vi "Basic NPL DS Write-Read external.vi"(5 "TimeOut Time (s)":dbl format="%.2f", 6 "error in (no error)":errorcluster, 7 "Server Mode":T2, 8 "Operation Mode":enum16{"Read", "Write", "Write/Read"}(ring), 9 "DataSocketCluster In":T1 {"TimeStamp" format="%.2f"}) -> (0 "error out":errorcluster, 2 "New Data":bool, 3 "DataSocketCluster Out":T1 {"TimeStamp" format="%.2f"})   [LabVIEW 2020]
uses:
  vi Mode external.ctl
  DataSocketCluster external.ctl
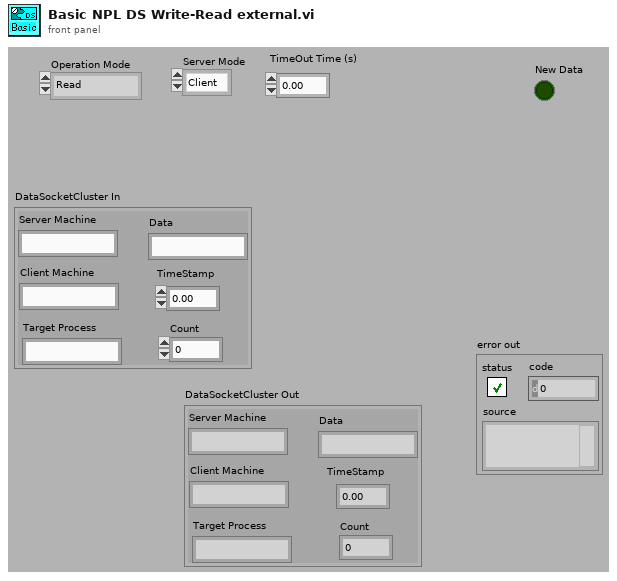
[diagram p1: front panel]
types:
  T1 = typedef "DataSocketCluster external.ctl" = cluster{"Server Machine":string, "Client Machine":string, "Data":string, "TimeStamp":dbl, "Count":i32, "Target Process":string}
  T2 = typedef "vi Mode external.ctl" = enum16{"Client", "Server"}
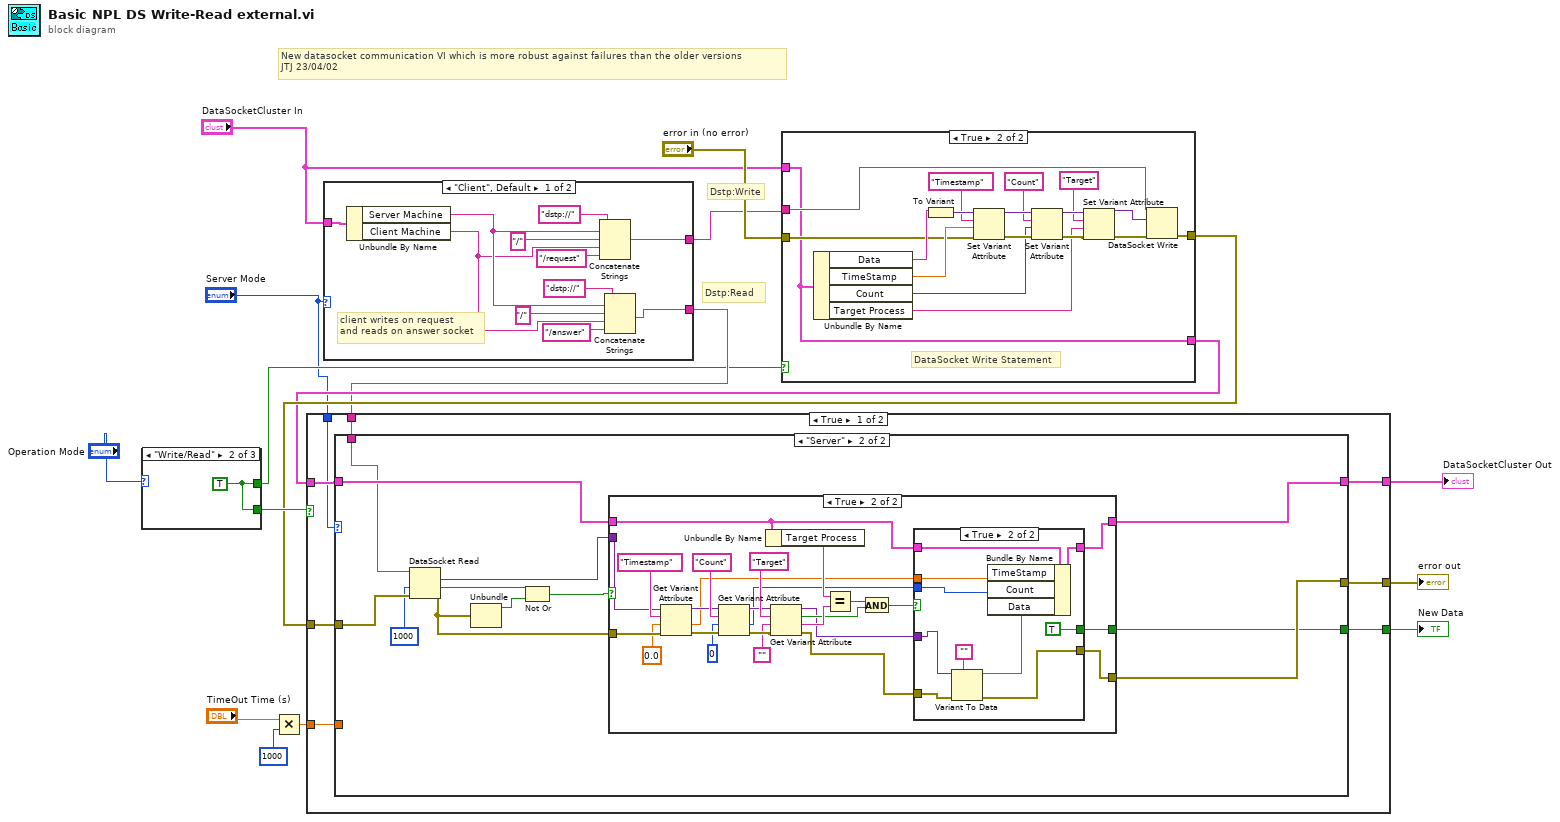
[diagram p0: block diagram]
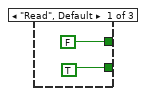
[diagram p2: hidden frame]
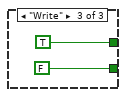
[diagram p3: hidden frame]
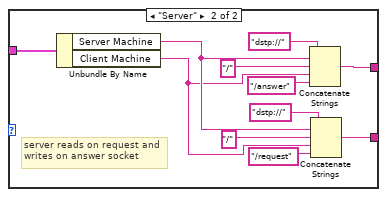
[diagram p5: hidden frame]
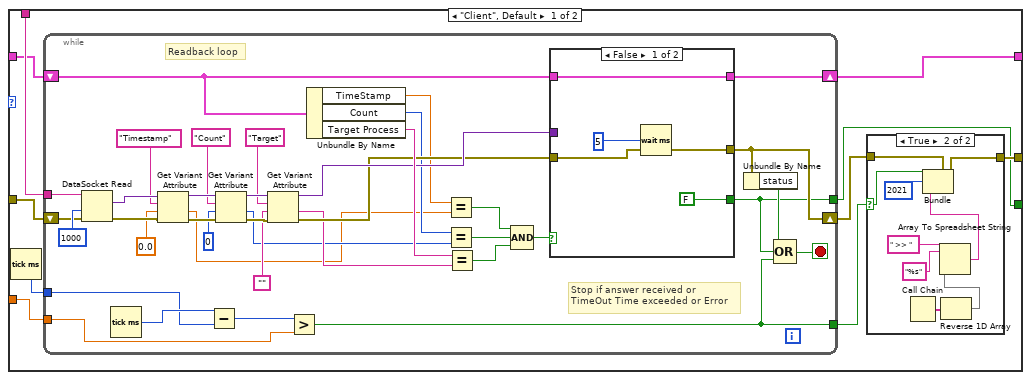
[diagram p6: hidden frame]
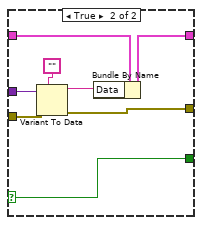
[diagram p7: hidden frame]
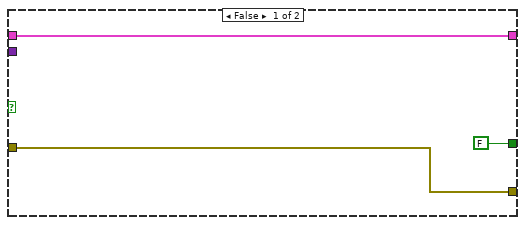
[diagram p9: hidden frame]
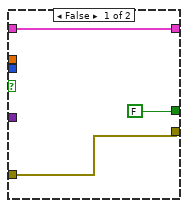
[diagram p10: hidden frame]
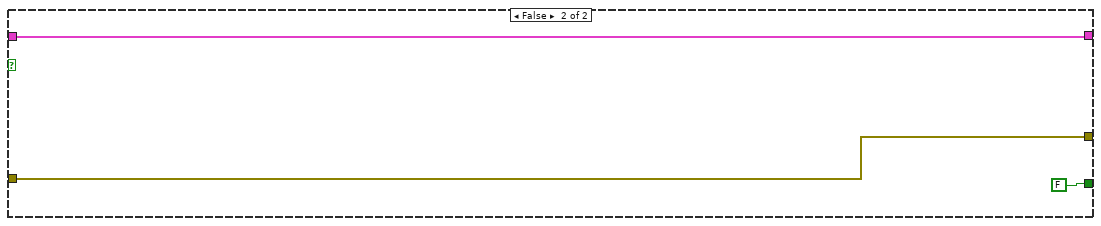
[diagram p11: hidden frame]
diagram:
  # "New datasocket communication VI which is more robust against failures than the older versions\nJTJ 23/04/02"
  # "Dstp:Read"
  # "Dstp:Write"
  n1 = case shown="\"Write/Read\"" "Operation Mode" {
    tunnel: [FALSE w19 TRUE] -> w5
    tunnel: [TRUE w19 FALSE] -> w14
    frame "Read", Default {
    }
    frame "Write/Read" {
      w19 = TRUE
    }
    frame "Write" {
    }
  }
  n2 = Multiply(x="TimeOut Time (s)", y=1000) -> (x*y=w6:dbl)
  n3 = case shown="\"Client\", Default" "Server Mode" {
    tunnel: "DataSocketCluster In" -> [w29 w43]
    tunnel: [w28 w39] -> w10
    tunnel: [w24 w35] -> w11
    frame "Client", Default {
      # "client writes on request\nand reads on answer socket"
      n4 = Unbundle By Name(w29) -> ("Server Machine"=w23:string, "Client Machine"=w22:string)
      n5 = Concatenate Strings("dstp://", w23, "/", w22, "/request") -> (w28:string)
      n6 = Concatenate Strings("dstp://", w23, "/", w22, "/answer") -> (w24:string)
    }
    frame "Server" {
      # "server reads on request and\nwrites on answer socket"
      n7 = Unbundle By Name(w43) -> ("Server Machine"=w34:string, "Client Machine"=w33:string)
      n8 = Concatenate Strings("dstp://", w34, "/", w33, "/answer") -> (w39:string)
      n9 = Concatenate Strings("dstp://", w34, "/", w33, "/request") -> (w35:string)
    }
  }
  n10 = case shown="True" w5 {
    tunnel: "error in (no error)" -> [w45 w49]
    tunnel: [w45 w48] -> w13
    tunnel: [w44 w46] -> w12
    tunnel: "DataSocketCluster In" -> [w44 w46]
    tunnel: w10 -> [_ w47]
    frame False {
    }
    frame True {
      # "DataSocket Write Statement"
      n11 = Unbundle By Name(w46) -> ("Data"=w53:string, "TimeStamp"=w52:dbl, "Count"=w51:i32, "Target Process"=w50:string)
      n12 = To Variant(anything=w53) -> (Variant=w63:variant)
      n13 = Set Variant Attribute(Variant=w63, name="Timestamp", value=w52, error in=w49) -> (Variant out=w62:variant, error out=w56:errorcluster)  [unwired: 1 out]
      n14 = Set Variant Attribute(Variant=w62, name="Count", value=w51, error in=w56) -> (Variant out=w61:variant, error out=w55:errorcluster)  [unwired: 1 out]
      n15 = Set Variant Attribute(Variant=w61, name="Target", value=w50, error in=w55) -> (Variant out=w57:variant, error out=w54:errorcluster)  [unwired: 1 out]
      n16 = DataSocket Write(8:w54, 10:w57, 11:w47) -> (0:w48:errorcluster)  [unwired: 1 in, 2 out]
    }
  }
  n17 = case shown="True" w14 {
    tunnel: w13 -> [w70 w196]
    tunnel: w11 -> [w71 _]
    tunnel: [w68 w197] -> w2
    tunnel: w6 -> [w69 _]
    tunnel: w12 -> [w67 w197]
    tunnel: [w66 w196] -> w9
    tunnel: "Server Mode" -> [w65 _]
    tunnel: [w64 FALSE] -> w4
    frame True {
      n18 = case shown="\"Server\"" w65 {
        tunnel: w71 -> [w81 w146]
        tunnel: w70 -> [w80 w148]
        tunnel: w69 -> [w78 _]
        tunnel: [w77 w143] -> w68
        tunnel: w67 -> [w76 w147]
        tunnel: [w73 w144] -> w66
        tunnel: [w72 w142] -> w64
        frame "Client", Default {
          n19 = Tick Count (ms)() -> (millisecond timer value=w79:u32)
          n20 = while {
            tunnel: [w83] -> w72
            tunnel: [w85] -> w75
            tunnel: w78 -> [w89]
            tunnel: w79 -> [w91]
            shift-left: w76 -> [w99]
            shift-right: [w98] -> w77
            shift-left: w80 -> [w108]
            shift-right: [w86] -> w74
            tunnel: w81 -> [w118]
            stop <- w87 stop-if-true
            # "Stop if answer received or\nTimeOut Time exceeded or Error"
            # "Readback loop"
            n21 = DataSocket Read(8:w108, 9:1000, 11:w118) -> (0:w111:errorcluster, 2:w115:variant)  [unwired: 2 in, 5 out]
            n22 = Tick Count (ms)() -> (millisecond timer value=w92:u32)
            n23 = Get Variant Attribute(Variant=w115, name="Timestamp", default value (empty Variant)=0.0, error in=w111) -> (duplicate Variant=w116:variant, value=w93:dbl, error out=w110:errorcluster)  [unwired: 1 out]
            n24 = Subtract(x=w92, y=w91) -> (x-y=w90:u32)
            n25 = Get Variant Attribute(Variant=w116, name="Count", default value (empty Variant)=0, error in=w110) -> (duplicate Variant=w117:variant, value=w94:i32, error out=w109:errorcluster)  [unwired: 1 out]
            n26 = Get Variant Attribute(Variant=w117, name="Target", default value (empty Variant)="", error in=w109) -> (duplicate Variant=w101:variant, value=w95:string, error out=w100:errorcluster)  [unwired: 1 out]
            n27 = Greater?(x=w90, y=w89) -> (0:w85:bool)
            n28 = Unbundle By Name(w99) -> ("TimeStamp"=w97:dbl, "Count"=w96:i32, "Target Process"=w104:string)
            n29 = Equal?(x=w97, y=w93) -> (x = y?=w82:bool)
            n30 = Equal?(x=w96, y=w94) -> (x = y?=w84:bool)
            n31 = Equal?(x=w104, y=w95) -> (x = y?=w103:bool)
            n32 = Compound Arithmetic op=AND(w82, w84, w103) -> (w102:bool)
            n33 = case shown="False" w102 {
              selector: w102 -> [_ w128]
              tunnel: w101 -> [_ w131]
              tunnel: w100 -> [w121 w130]
              tunnel: [FALSE w128] -> w83
              tunnel: [w121 w127] -> w86
              tunnel: w99 -> [w120 w126]
              tunnel: [w120 w125] -> w98
              frame False {
                n34 = Wait (ms)(milliseconds to wait=5) -> ()  [unwired: 1 out]
              }
              frame True {
                n35 = Variant To Data(error in=w130, type="", Variant=w131) -> (data=w124:string, error out=w127:errorcluster)
                n36 = Bundle By Name(cluster=w126, "Data"=w124) -> (w125:T1)
              }
            }
            n37 = Unbundle By Name(w86) -> ("status"=w88:bool)
            n38 = Compound Arithmetic op=OR(w88, w83, w85) -> (w87:bool)
          }
          n39 = case shown="True" w75 {
            selector: w75 -> [_ w139]
            tunnel: w74 -> [w132 w141]
            tunnel: [w132 w140] -> w73
            frame False {
            }
            frame True {
              n40 = Call Chain() -> (call chain=w137:string[])
              n41 = Reverse 1D Array(array=w137) -> (reversed array=w134:string[])
              n42 = Array To Spreadsheet String(delimiter (Tab)=" >> ", array=w134, 3:"%s" ("format string")) -> (spreadsheet string=w133:string)
              n43 = Bundle(cluster=w141, "status"=w139, "code"=2021, "source"=w133) -> (w140:errorcluster)
            }
          }
        }
        frame "Server" {
          n44 = DataSocket Read(8:w148, 9:1000, 11:w146) -> (0:w152:errorcluster, 1:w151:bool, 2:w153:variant)  [unwired: 2 in, 4 out]
          n45 = Unbundle(w152) -> ("status"=w150:bool)  [unwired: 2 out]
          n46 = Not Or(1:w150, 2:w151) -> (0:w149:bool)
          n47 = case shown="True" w149 {
            tunnel: w147 -> [w154 w159]
            tunnel: w153 -> [_ w174]
            tunnel: w152 -> [w156 w173]
            tunnel: [w156 w160] -> w144
            tunnel: [FALSE w162] -> w142
            tunnel: [w154 w158] -> w143
            frame False {
            }
            frame True {
              n48 = Get Variant Attribute(Variant=w174, name="Timestamp", default value (empty Variant)=0.0, error in=w173) -> (duplicate Variant=w175:variant, value=w164:dbl, error out=w180:errorcluster)  [unwired: 1 out]
              n49 = Get Variant Attribute(Variant=w175, name="Count", default value (empty Variant)=0, error in=w180) -> (duplicate Variant=w176:variant, value=w163:i32, error out=w181:errorcluster)  [unwired: 1 out]
              n50 = Unbundle By Name(w159) -> ("Target Process"=w168:string)
              n51 = Get Variant Attribute(Variant=w176, name="Target", default value (empty Variant)="", error in=w181) -> (duplicate Variant=w161:variant, found=w166:bool, value=w169:string, error out=w157:errorcluster)
              n52 = Equal?(x=w168, y=w169) -> (x = y?=w167:bool)
              n53 = And(x=w167, y=w166) -> (x .and. y?=w165:bool)
              n54 = case shown="True" w165 {
                tunnel: w159 -> [w183 w190]
                tunnel: w164 -> [_ w194]
                tunnel: w163 -> [_ w193]
                tunnel: [FALSE TRUE] -> w162
                tunnel: w161 -> [_ w189]
                tunnel: [w182 w187] -> w160
                tunnel: [w183 w192] -> w158
                tunnel: w157 -> [w182 w188]
                frame False {
                }
                frame True {
                  n55 = Variant To Data(error in=w188, type="", Variant=w189) -> (data=w186:string, error out=w187:errorcluster)
                  n56 = Bundle By Name(cluster=w190, "TimeStamp"=w194, "Count"=w193, "Data"=w186) -> (w192:T1)
                }
              }
            }
          }
        }
      }
    }
    frame False {
    }
  }
  "error out" <- w9
  "New Data" <- w4
  "DataSocketCluster Out" <- w2
